vi "Delay_H_LOGtest.vi"(8 "error in":errorcluster, 11 "ATE Switches":T1) -> (0 "Switch Errors":errorcluster, 3 "ATE Switch Status":T2={"Reversing Switch "=TRUE, "IO Switch #1"=TRUE, "IO Switch #2"=TRUE, "Signal Out"=TRUE, "Signal Source"=TRUE, "Power Meter"=TRUE, "Amp By Pass"=TRUE})   [LabVIEW 2009]
panel:
  out "ATE SWITCH SETTINGS":T1
  in  "Delay Line Control":bool
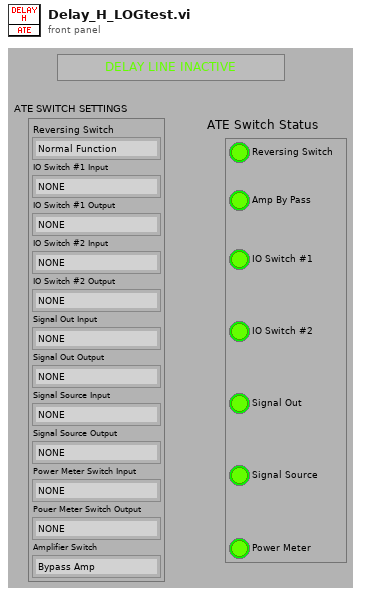
[diagram p1: front panel]
types:
  T1 = cluster{"Reversing Switch":enum16{"Normal Function", "Reversing Function"}, "IO Switch #1 Input":enum16{"NONE", "AHR (J2)", "Splitter", "Signal Out Switch (S3)", "Reversing Switch", "Power Meter Switch"}, "IO Switch #1 Output":enum16{"NONE", "AHR (J2)", "Delay Device (S4)", "Power Meter Switch (S5)", "Reversing Switch"}, "IO Switch #2 Input":enum16{"NONE", "AVR (J3)", "Splitter", "Signal Out Switch (S3)", " 2W Term (TM1)", "Reversing Switch", "Power Meter Switch"}, "IO Switch #2 Output":enum16{"NONE", "AVR (J3)", "Signal Out Switch (S3)", "Power Meter Switch (S5)", "Reversing Switch", "2W Term (TM1)"}, "Signal Out Input":enum16{"NONE", "Amp Bypass Switch (S6)", "IO Switch #1 (S1)", "IO Switch #2 (S2)", "2W Term (TM3)"}, "Signal Out Output":enum16{"NONE", "2 Watt Term (TM3)", "Splitter", "Power Meter Switch (S5)"}, "Signal Source Input":enum16{"NONE", "Delay Device", "Signal Generator (J7)", "Inside Noise Box NF (J5)", "2W Term (TM3)"}, "Signal Source Output":enum16{"NONE", "Amp Bypass Switch", "Test Pulse Generator", "Power Meter Switch (S5)"}, "Power Meter Switch Input":enum16{"NONE", "IO Switch #1 (S1)", "Signal Source Switch (S4)", "Signal Out Switch (S3)", "IO Switch #2 (S2)", "TXH-TXV Switch (J8)"}, "Pouer Meter Switch Output":enum16{"NONE", "Power Meter (J6)", "IO Switch # 1", "IO Switch # 2"}, "Amplifier Switch":enum16{"Bypass Amp", "Include Amp"}}
  T2 = cluster{"Reversing Switch ":bool, "IO Switch #1":bool, "IO Switch #2":bool, "Signal Out":bool, "Signal Source":bool, "Power Meter":bool, "Amp By Pass":bool}
  T3 = enum16{"NONE", "AHR (J2)", "Splitter", "Signal Out Switch (S3)", "Reversing Switch", "Power Meter Switch"}
  T4 = enum16{"NONE", "AHR (J2)", "Delay Device (S4)", "Power Meter Switch (S5)", "Reversing Switch"}
  T5 = enum16{"NONE", "AVR (J3)", "Splitter", "Signal Out Switch (S3)", " 2W Term (TM1)", "Reversing Switch", "Power Meter Switch"}
  T6 = enum16{"NONE", "AVR (J3)", "Signal Out Switch (S3)", "Power Meter Switch (S5)", "Reversing Switch", "2W Term (TM1)"}
  T7 = enum16{"NONE", "Amp Bypass Switch (S6)", "IO Switch #1 (S1)", "IO Switch #2 (S2)", "2W Term (TM3)"}
  T8 = enum16{"NONE", "2 Watt Term (TM3)", "Splitter", "Power Meter Switch (S5)"}
  T9 = enum16{"NONE", "Delay Device", "Signal Generator (J7)", "Inside Noise Box NF (J5)", "2W Term (TM3)"}
  T10 = enum16{"NONE", "Amp Bypass Switch", "Test Pulse Generator", "Power Meter Switch (S5)"}
  T11 = enum16{"NONE", "IO Switch #1 (S1)", "Signal Source Switch (S4)", "Signal Out Switch (S3)", "IO Switch #2 (S2)", "TXH-TXV Switch (J8)"}
  T12 = enum16{"NONE", "Power Meter (J6)", "IO Switch # 1", "IO Switch # 2"}
  T13 = cluster{"Verfied":bool, "Verfied":bool, "Verfied":bool, "Verfied":bool, "Verfied":bool, "Verfied":bool, "Verfied":bool}
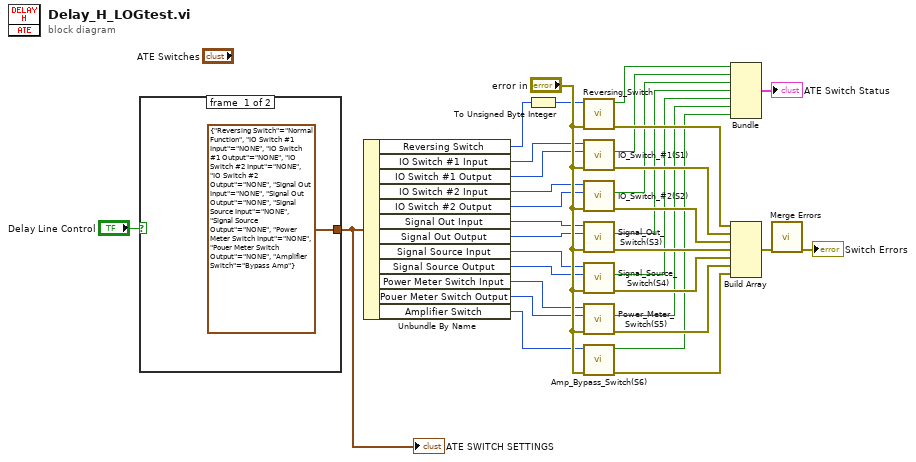
[diagram p0: block diagram]
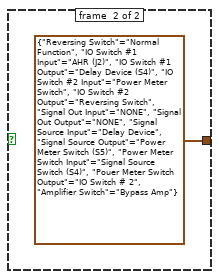
[diagram p2: hidden frame]
diagram:
  n1 = case shown="True" "Delay Line Control" {
    tunnel: [T1 {"Reversing Switch"=enum."Normal Function", "IO Switch #1 Input"=enum."NONE", "IO Switch #1 Output"=enum."NONE", "IO Switch #2 Input"=enum."NONE", "IO Switch #2 Output"=enum."NONE", "Signal Out Input"=enum."NONE", "Signal Out Output"=enum."NONE", "Signal Source Input"=enum."NONE", "Signal Source Output"=enum."NONE", "Power Meter Switch Input"=enum."NONE", "Pouer Meter Switch Output"=enum."NONE", "Amplifier Switch"=enum."Bypass Amp"} ("ATE Switches 2") T1 {"Reversing Switch"=enum."Normal Function", "IO Switch #1 Input"=enum."AHR (J2)", "IO Switch #1 Output"=enum."Delay Device (S4)", "IO Switch #2 Input"=enum."Power Meter Switch", "IO Switch #2 Output"=enum."Reversing Switch", "Signal Out Input"=enum."NONE", "Signal Out Output"=enum."NONE", "Signal Source Input"=enum."Delay Device", "Signal Source Output"=enum."Power Meter Switch (S5)", "Power Meter Switch Input"=enum."Signal Source Switch (S4)", "Pouer Meter Switch Output"=enum."IO Switch # 2", "Amplifier Switch"=enum."Bypass Amp"} ("ATE Switches 2")] -> w2
    frame #0 {
    }
    frame #1 {
    }
  }
  "ATE SWITCH SETTINGS" <- w2
  n2 = Unbundle By Name(w2) -> ("Reversing Switch"=w23:enum16{"Normal Function", "Reversing Function"}, "IO Switch #1 Input"=w20:T3, "IO Switch #1 Output"=w13:T4, "IO Switch #2 Input"=w14:T5, "IO Switch #2 Output"=w15:T6, "Signal Out Input"=w16:T7, "Signal Out Output"=w17:T8, "Signal Source Input"=w18:T9, "Signal Source Output"=w4:T10, "Power Meter Switch Input"=w19:T11, "Pouer Meter Switch Output"=w21:T12, "Amplifier Switch"=w22:enum16{"Bypass Amp", "Include Amp"})
  n3 = To Unsigned Byte Integer(number=w23) -> (unsigned 8bit integer=w1:u8)
  n4 = call "Reversing_Switch.vi"("error in"="error in", "Reversing Switch Function"=w1) -> ("error out"=w24:errorcluster, "Verfied"=w11:bool)  [unwired: 8 in]
  n5 = call "IO_Switch_#1(S1).vi"("error in"="error in", "Output"=w13, "Input"=w20) -> ("error out"=w25:errorcluster, "Verfied"=w10:bool)  [unwired: 6 in, 1 out]
  n6 = call "IO_Switch_#2(S2).vi"("error in"="error in", "Output"=w15, "Input"=w14) -> ("error out"=w26:errorcluster, "Verfied"=w9:bool)  [unwired: 6 in, 1 out]
  n7 = call "Signal_Out_Switch(S3).vi"("error in"="error in", "Output"=w17, "Input"=w16) -> ("error out"=w28:errorcluster, "Verfied"=w8:bool)  [unwired: 6 in, 1 out]
  n8 = call "Signal_Source_Switch(S4).vi"("error in"="error in", "Output"=w4, "Input"=w18) -> ("error out"=w29:errorcluster, "Verfied"=w7:bool)  [unwired: 6 in, 1 out]
  n9 = call "Power_Meter_Switch(S5).vi"("error in"="error in", "Output"=w21, "Input"=w19) -> ("error out"=w30:errorcluster, "Verfied"=w6:bool)  [unwired: 6 in, 1 out]
  n10 = call "Amp_Bypass_Switch(S6).vi"("error in"="error in", "AMP Function"=w22) -> ("error out"=w31:errorcluster, "Verfied"=w5:bool)  [unwired: 8 in]
  n11 = Bundle("Verfied"=w11, "Verfied"=w10, "Verfied"=w9, "Verfied"=w8, "Verfied"=w7, "Verfied"=w6, "Verfied"=w5) -> (→"ATE Switch Status":T13)  [unwired: 1 in]
  n12 = Build Array(w24, w25, w26, w28, w29, w30, w31) -> (w27:errorcluster[])
  n13 = call <vilib>:"Merge Errors.vi"("error array in"=w27) -> ("error out"=→"Switch Errors":errorcluster)  [unwired: 6 in]
